vi "getOutputWithTemperature.vi"(8 "error in (no error)":errorcluster, 10 "Reading Option (0: Latest)":i32, 11 "Electrometer in":refnum<class "Electrometer.lvclass">) -> (0 "error out":errorcluster, 1 "Temperature":string, 2 "READings":string, 3 "Electrometer out":refnum<class "Electrometer.lvclass">)   [LabVIEW 2016, in "Electrometer.lvclass"]
uses:
  Electrometer.lvclass
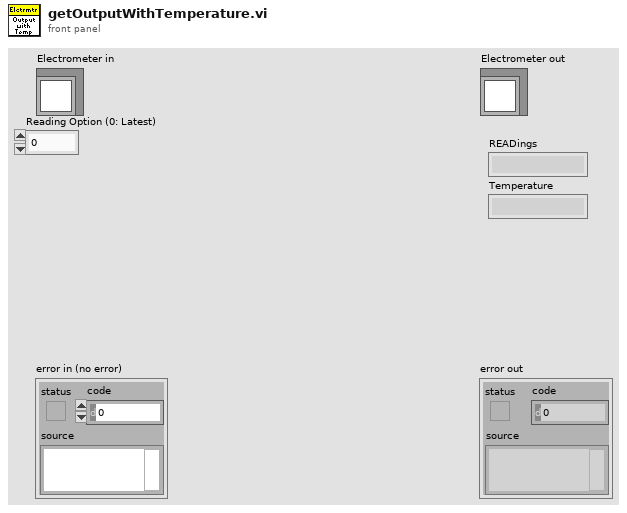
[diagram p1: front panel]
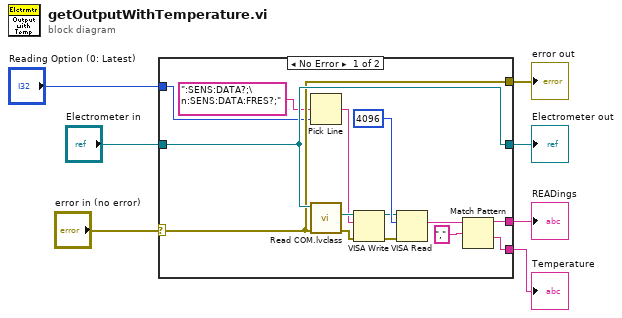
[diagram p0: block diagram]
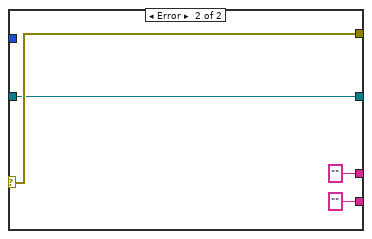
[diagram p2: hidden frame]
diagram:
  n1 = case shown="No Error" "error in (no error)" {
    selector: "error in (no error)" -> [w18 w25]
    tunnel: [w18 w25] -> w6
    tunnel: [w19 w24] -> w4
    tunnel: "Electrometer in" -> [w19 w24]
    tunnel: "Reading Option (0: Latest)" -> [w13 _]
    tunnel: [w9 "" ("read buffer")] -> w2
    tunnel: [w8 "" ("read buffer")] -> w1
    frame No Error {
      n2 = Pick Line(multi-line string=":SENS:DATA?;\n:SENS:DATA:FRES?;", line index=w13) -> (output string=w14:string)  [unwired: 1 in]
      n3 = call "Read COM.lvclass.vi"("error in (no error)"=w18, "Electrometer in"=w19) -> ("error out"=w17:errorcluster, "VISA"=w15:refnum<visa-resource-name>)  [unwired: 7 in, 1 out]
      n4 = VISA Write(VISA resource name=w15, write buffer=w14, error in (no error)=w17) -> (VISA resource name out=w20:refnum<visa-resource-name>, error out=w16:errorcluster)  [unwired: 1 out]
      n5 = VISA Read(VISA resource name=w20, byte count=u32 4096, error in (no error)=w16) -> (read buffer=w10:string)  [unwired: 3 out]
      n6 = Match Pattern(string=w10, regular expression="," ("search string/char (-)")) -> (before substring=w9:string, after substring=w8:string)  [unwired: 1 in, 2 out]
    }
    frame Error {
    }
  }
  "error out" <- w6
  "Electrometer out" <- w4
  "READings" <- w2
  "Temperature" <- w1
